vi "dosimat_fill_&_relay_vent.vi"(2 "relay session in":T3={"VISA resource out"="COM12", "error out"={"status"=FALSE, "code"=0, "source"=""}}, 3 "Dosimat In":T1={"Dosimat Port in"="COM1", "Error in"={"status"=FALSE, "code"=0, "source"=""}}) -> (0 "relay session out":T3={"VISA resource out"="COM12", "error out"={"status"=FALSE, "code"=0, "source"=""}}, 1 "Dosimat Out":T2={"Dosimat Port out"="COM1", "Error out"={"status"=FALSE, "code"=0, "source"=""}})   [LabVIEW 2010]
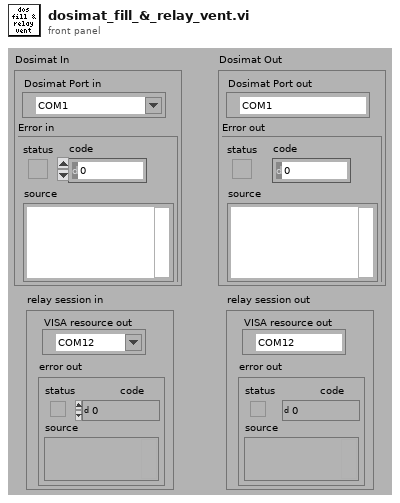
[diagram p1: front panel]
types:
  T1 = cluster{"Dosimat Port in":refnum<visa-resource-name>, "Error in":errorcluster}
  T2 = cluster{"Dosimat Port out":refnum<visa-resource-name>, "Error out":errorcluster}
  T3 = cluster{"VISA resource out":refnum<visa-resource-name>, "error out":errorcluster}
  T4 = cluster{"Dosimat Port Out":refnum<visa-resource-name>, "error out":errorcluster}
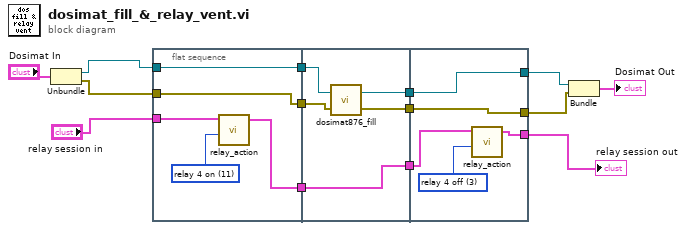
[diagram p0: block diagram]
diagram:
  n1 = Unbundle("Dosimat In") -> ("Dosimat Port in"=w6:refnum<visa-resource-name>, "Error in"=w5:errorcluster)
  n2 = flat-sequence {
    tunnel: "relay session in" -> [w18]
    tunnel: [w17] -> w12
    tunnel: w6 -> [w16]
    tunnel: [w16] -> w8
    tunnel: [w15] -> w7
    tunnel: w5 -> [w15]
    tunnel: [w24] -> w13
    tunnel: w12 -> [w24]
    tunnel: [w23] -> w10
    tunnel: [w22] -> w9
    tunnel: w8 -> [w21]
    tunnel: w7 -> [w20]
    tunnel: w13 -> [w28]
    tunnel: [w27] -> w11
    tunnel: [w26] -> w3
    tunnel: w10 -> [w26]
    tunnel: [w25] -> w2
    tunnel: w9 -> [w25]
    frame #0 {
      w19 = u8 11 items=["relay 1 on"=8, "relay 2 on"=9, "relay 3 on"=10, "relay 4 on"=11, "relay 1 off"=0, "relay 2 off"=1, "relay 3 off"=2, "relay 4 off"=3, "OpenAll"=30, "CloseAll"=29] ("Action")
      n3 = call "relay_action.vi"("relay session in"=w18, "Action"=w19) -> ("relay session out"=w17:T3)  [unwired: 6 in]
    }
    frame #1 {
      n4 = call "dosimat876_fill.vi"("error in"=w20, "Dosimat Port In"=w21) -> ("error out"=w22:errorcluster, "Dosimat Port Out"=w23:refnum<visa-resource-name>)
    }
    frame #2 {
      w29 = u8 3 items=["relay 1 on"=8, "relay 2 on"=9, "relay 3 on"=10, "relay 4 on"=11, "relay 1 off"=0, "relay 2 off"=1, "relay 3 off"=2, "relay 4 off"=3, "OpenAll"=30, "CloseAll"=29] ("Action")
      n5 = call "relay_action.vi"("relay session in"=w28, "Action"=w29) -> ("relay session out"=w27:T3)  [unwired: 6 in]
    }
  }
  n6 = Bundle("Dosimat Port Out"=w3, "error out"=w2) -> (→"Dosimat Out":T4)  [unwired: 1 in]
  "relay session out" <- w11
